vi "UDCStop.vi"(2 "Error In":errorcluster) -> (0 "Error Out":errorcluster)   [LabVIEW 2020, in "niceiplib.lvlib"]
doc: "This API is used to stop and commit the Usage Data Collection. It is advised to call this API at the end of the Application exit."
uses:
  <vilib>/UDC/niceiplib.lvlib
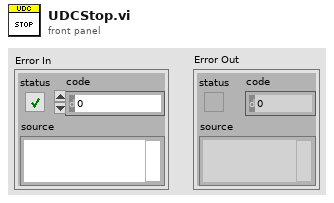
[diagram p1: front panel]
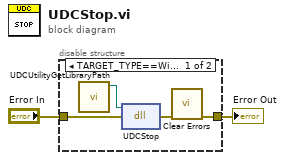
[diagram p0: block diagram]
diagram:
  n1 = disable-structure shown="TARGET_TYPE==Windows" {
    disable-tunnel: "Error In" -> [w6 w7]
    disable-tunnel: [w4 w7] -> w1
    frame condition #0 (active) {
      n2 = call <vilib>:"UDCUtilityGetLibraryPath.vi"() -> ("Library Path"=w3:path)  [unwired: 11 in]
      n3 = dll-call lib="C:/2013LabVIEWCode/dist/vi.lib/UDC/niceiplib.*" fn="UDCStop"(path in=w3, error in=w6) -> (error out=w5:errorcluster)  [unwired: 2 in, 1 out]
      n4 = call <vilib>:"Clear Errors.vi"("error in (no error)"=w5) -> ("error out"=w4:errorcluster)  [unwired: 5 in, 1 out]
    }
    frame condition #1 {
    }
  }
  "Error Out" <- w1
